vi "TriggerRotationAcquire.vi"(0 "Microscope in":refnum<class "Microscope.lvclass">, 1 "Trigger":bool, 11 "error in (no error)":errorcluster) -> (4 "Microscope out":refnum<class "Microscope.lvclass">, 15 "error out":errorcluster)   [LabVIEW 2012, in "Microscope.lvclass"]
uses:
  classes/Microscope.lvclass
  classes/Microscope.lvclass/Microscope.ctl
  RotationProgram/Event/MainEvents.ctl
  RotationProgram/Global/RotationGlobal.vi
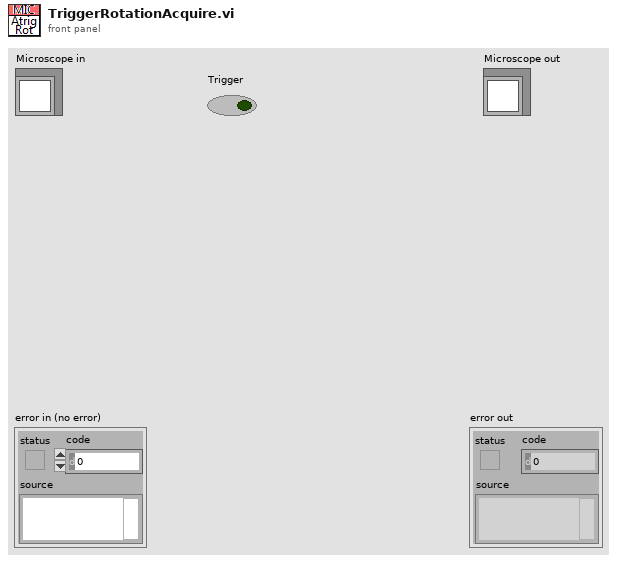
[diagram p1: front panel]
types:
  T1 = typedef "MainEvents.ctl" = enum16{"Initialize", "Initialize Angle Scan", "Acquire Angle Scan", "Move to Zero", "Home", "Send Request", "Move Relative Negative", "Move Relative", "Optimize", "Move Absolute", "Calibrate Angle-Stage", "Restore Sync Parameters", "Sync Formula", "Sync Data", "Sync Data Shotgun", "Restore Booleans", "Disable Buttons", "Enable Buttons"}
  T2 = typedef "ScanMode.ctl" = enum16{"None", "Continuous", "Point Scan (CH3 cursor)", "Point Scan Move (CH3 cursor)", "Grab", "Grab Move Stage", "Grab Move Z-stage", "Cont. Move Z-stage", "Spec Move Stage", "Spec Move Cont", "Surf Calib"}
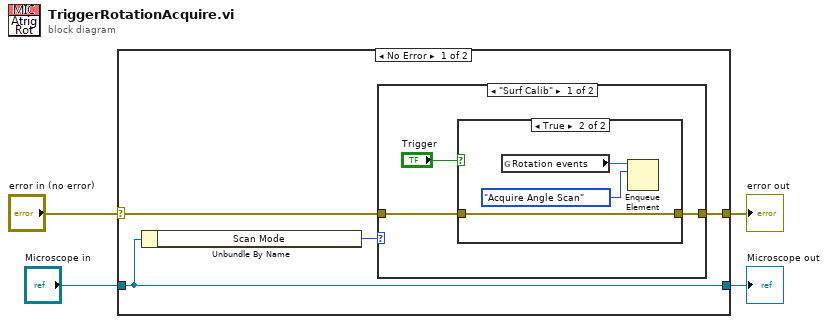
[diagram p0: block diagram]
diagram:
  n1 = case shown="No Error" "error in (no error)" {
    selector: "error in (no error)" -> [w8 w17]
    tunnel: [w7 w17] -> w3
    tunnel: [w5 w16] -> w1
    tunnel: "Microscope in" -> [w5 w16]
    frame No Error {
      n2 = Unbundle By Name(w5) -> ("Scan Mode"=w6:T2)
      n3 = case shown="\"Surf Calib\"" w6 {
        tunnel: w8 -> [w11 w15]
        tunnel: [w10 w15] -> w7
        frame "Surf Calib" {
          n4 = case shown="True" "Trigger" {
            tunnel: w11 -> [_ w14]
            tunnel: [_ w14] -> w10
            frame False {
            }
            frame True {
              n5 = global read "RotationGlobal.vi" "Rotation events"() -> (w13:refnum<queue>)
              n6 = Enqueue Element(queue=w13, element=MainEvents."Acquire Angle Scan") -> ()  [unwired: 2 in, 3 out]
            }
          }
        }
        frame "None", Default {
        }
      }
    }
    frame Error {
    }
  }
  "error out" <- w3
  "Microscope out" <- w1
